vi "ChangeNotification.vi"(0 "reference in":refnum<class "WeatherStation.lvclass">, 2 "WeatherData":T1, 5 "error in (no error)":errorcluster) -> (14 "reference out":refnum<class "WeatherStation.lvclass">, 19 "error out":errorcluster)   [LabVIEW 2010, in "WeatherStation.lvclass"]
uses:
  WeatherStation.lvclass
  WeatherData.ctl
  Observer_class/Observer.lvclass
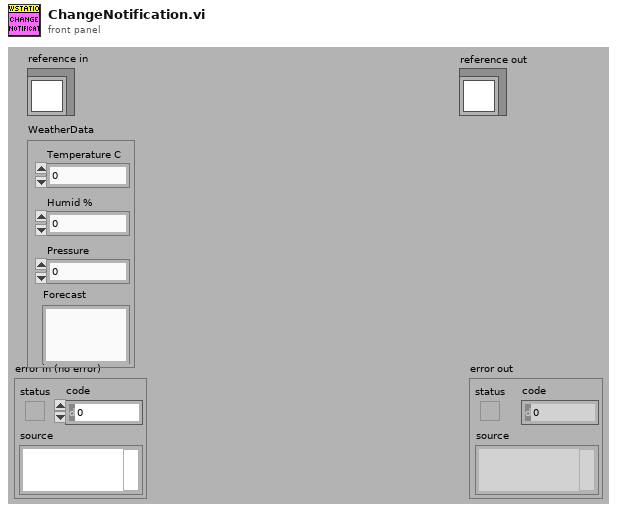
[diagram p1: front panel]
types:
  T1 = typedef "WeatherData.ctl" = cluster{"Temperature C":dbl, "Humid %":dbl, "Pressure":dbl, "Forecast":string}
  T2 = typedef "WeatherStation.lvclass/ObjectAttributes.ctl" = cluster{"WeatherData":T1, "Observers":refnum<class "Observer.lvclass">[]}
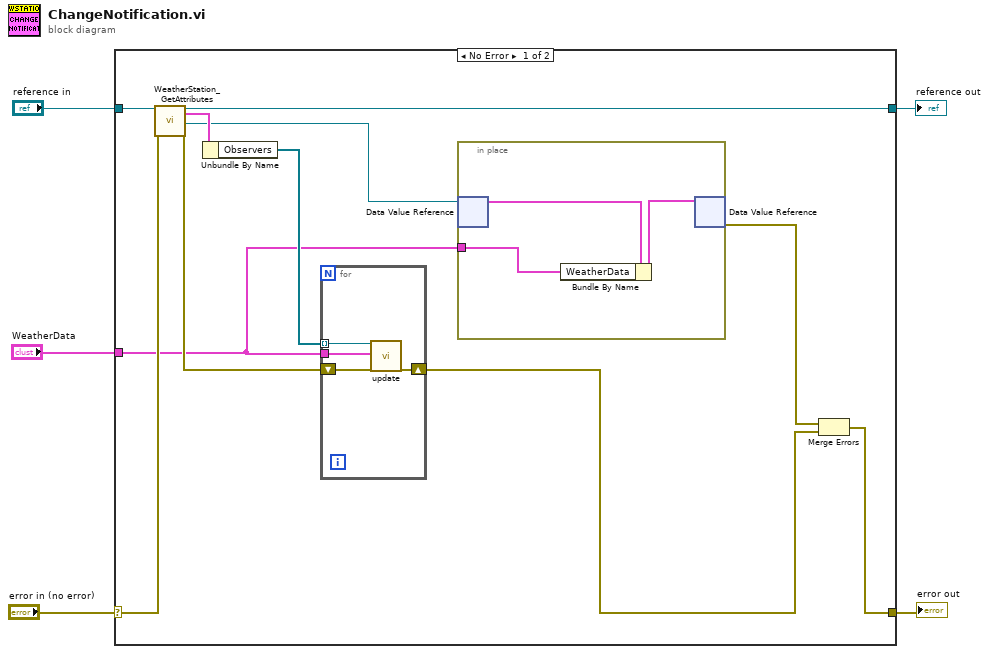
[diagram p0: block diagram]
diagram:
  n1 = case shown="No Error" "error in (no error)" {
    selector: "error in (no error)" -> [w16 w25]
    tunnel: [w6 w25] -> w4
    tunnel: [w13 w24] -> w2
    tunnel: "reference in" -> [w14 w24]
    tunnel: "WeatherData" -> [w8 _]
    frame No Error {
      n2 = call "WeatherStation_GetAttributes.vi"("reference in"=w14, "error in (no error)"=w16) -> ("reference out"=w13:refnum<class "WeatherStation.lvclass">, "Data"=w15:T2, "DataRef"=w9:refnum<data-value>, "error out"=w11:errorcluster)  [unwired: 14 in]
      n3 = Unbundle By Name(w15) -> ("Observers"=w12:refnum<class "Observer.lvclass">[])
      n4 = for {
        tunnel: w12 -> [w23] mode=indexing
        shift-right: [w21] -> w7
        shift-left: w11 -> [w22]
        tunnel: w8 -> [w20]
        n5 = call-dynamic "update.vi"("reference in"=w23, "WeatherData"=w20, "error in (no error)"=w22) -> ("error out"=w21:errorcluster)  [unwired: 15 in, 1 out]
      }
      n6 = in-place {
        in-place-border: w8 -> [w17]
        n7 = in-place-dvr #1(w9) -> (w19:T2)  [unwired: 1 out]
        n8 = Bundle By Name(cluster=w19, "WeatherData"=w17) -> (w18:T2)
        n9 = in-place-dvr #1(w18) -> (w10:errorcluster)  [unwired: 1 out]
      }
      n10 = Merge Errors(w10, w7) -> (w6:errorcluster)
    }
    frame Error {
    }
  }
  "error out" <- w4
  "reference out" <- w2
